vi "Scan From String, Format Into String part 4.vi"() -> ()   [LabVIEW 2020]
panel:
  out "resulting string":string
  in  "input 1":dbl
  in  "input string":string
  out "output 1":dbl
  # "Part 4"
  # "Scan From String, Format Into String"
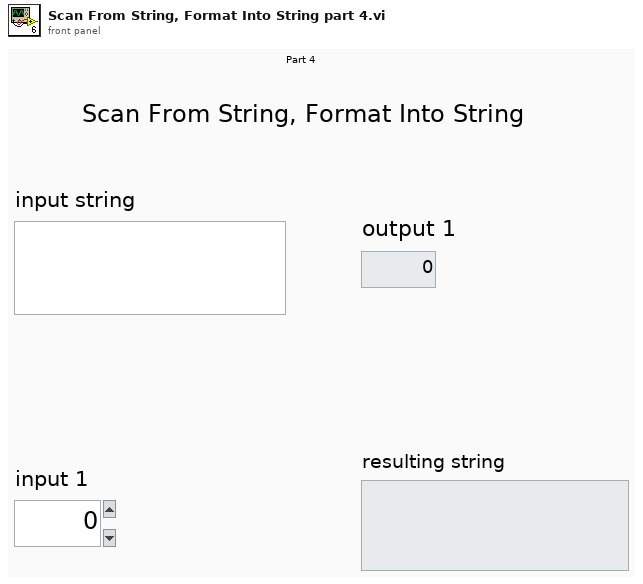
[diagram p1: front panel]
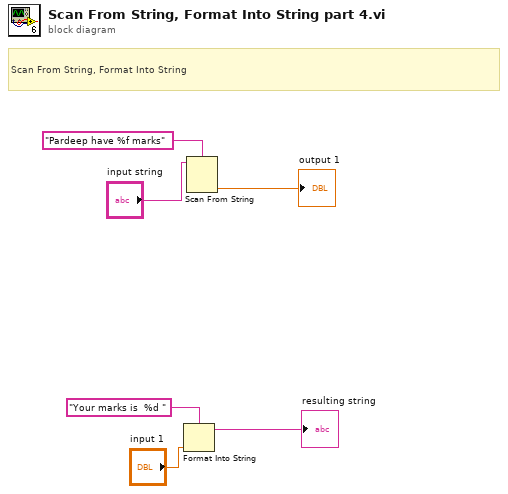
[diagram p0: block diagram]
diagram:
  # "Scan From String, Format Into String"
  n1 = Format Into String "Format Into String"(format string="Your marks is  %d ", "input 1") -> (resulting string=→"resulting string":string)  [unwired: 2 in, 1 out]
  n2 = Scan From String "Scan From String"(format string="Pardeep have %f marks", input string="input string") -> (output 1=→"output 1":dbl)  [unwired: 3 in, 3 out]
